vi "think_and_act.vi"(8 "error in (no error)":errorcluster, 9 "antState":T1, 10 "pieceOfWorld":T4[][](array[typedef]), 11 "Igor in":refnum<class "Igor.lvclass">) -> (0 "error out":errorcluster, 2 "action":T2, 3 "Igor out":refnum<class "Igor.lvclass">)   [LabVIEW 2015, in "Igor.lvclass"]
doc: "Ant thinks and chooses action\nCreated by Artem Shevelev\nshevelev.pro\nartem@shevelev.pro\nLabVIEW Portal: https://labviewportal.org/memberlist.php?mode=viewprofile&u=2340"
uses:
  Igor.lvclass
  actors/world/typedefs/worldCell_cluster.ctl
  actors/world/typedefs/markValue_cluster.ctl
  actors/world/typedefs/markValue.ctl
  actors/world/typedefs/markVolume.ctl
  actors/world/typedefs/amountOfFood.ctl
  actors/world/typedefs/anthillType_enum.ctl
  ant_base/action_cluster.ctl
  ant_base/actionType_enum.ctl
  ant_base/antState_cluster.ctl
  ant_base/ant_base.lvclass/ant_base.ctl
  ant_base/memory_limit_const.vi
  moving/move_forvard.vi
  moving/move_back.vi
  ant_base/ant_base.lvclass
  actors/world/world.lvlib
panel:
  out "Array":i32[][](array[numeric])
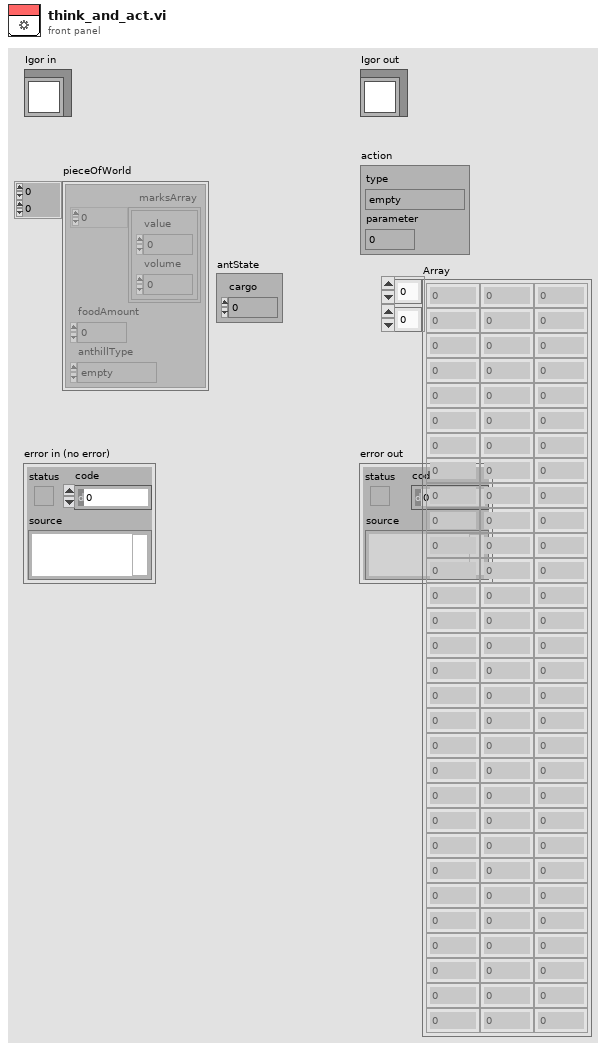
[diagram p1: front panel]
types:
  T1 = typedef "ant_base.lvclass/antState_cluster.ctl" = cluster{"cargo":u8}
  T2 = typedef "ant_base.lvclass/action_cluster.ctl" = cluster{"type":T3, "parameter":dbl}
  T3 = typedef "ant_base.lvclass/actionType_enum.ctl" = enum8{"empty", "move", "take", "put", "mark"}
  T4 = typedef "world.lvlib/worldCell_cluster.ctl" = cluster{"marksArray":T5[], "foodAmount":T8, "anthillType":T9}
  T5 = typedef "world.lvlib/markValue_cluster.ctl" = cluster{"value":T6, "volume":T7}
  T6 = typedef "world.lvlib/markValue.ctl" = u8
  T7 = typedef "world.lvlib/markVolume.ctl" = u16
  T8 = typedef "world.lvlib/amountOfFood.ctl" = i32
  T9 = typedef "world.lvlib/anthillType_enum.ctl" = enum16{"empty", "own", "rival"}
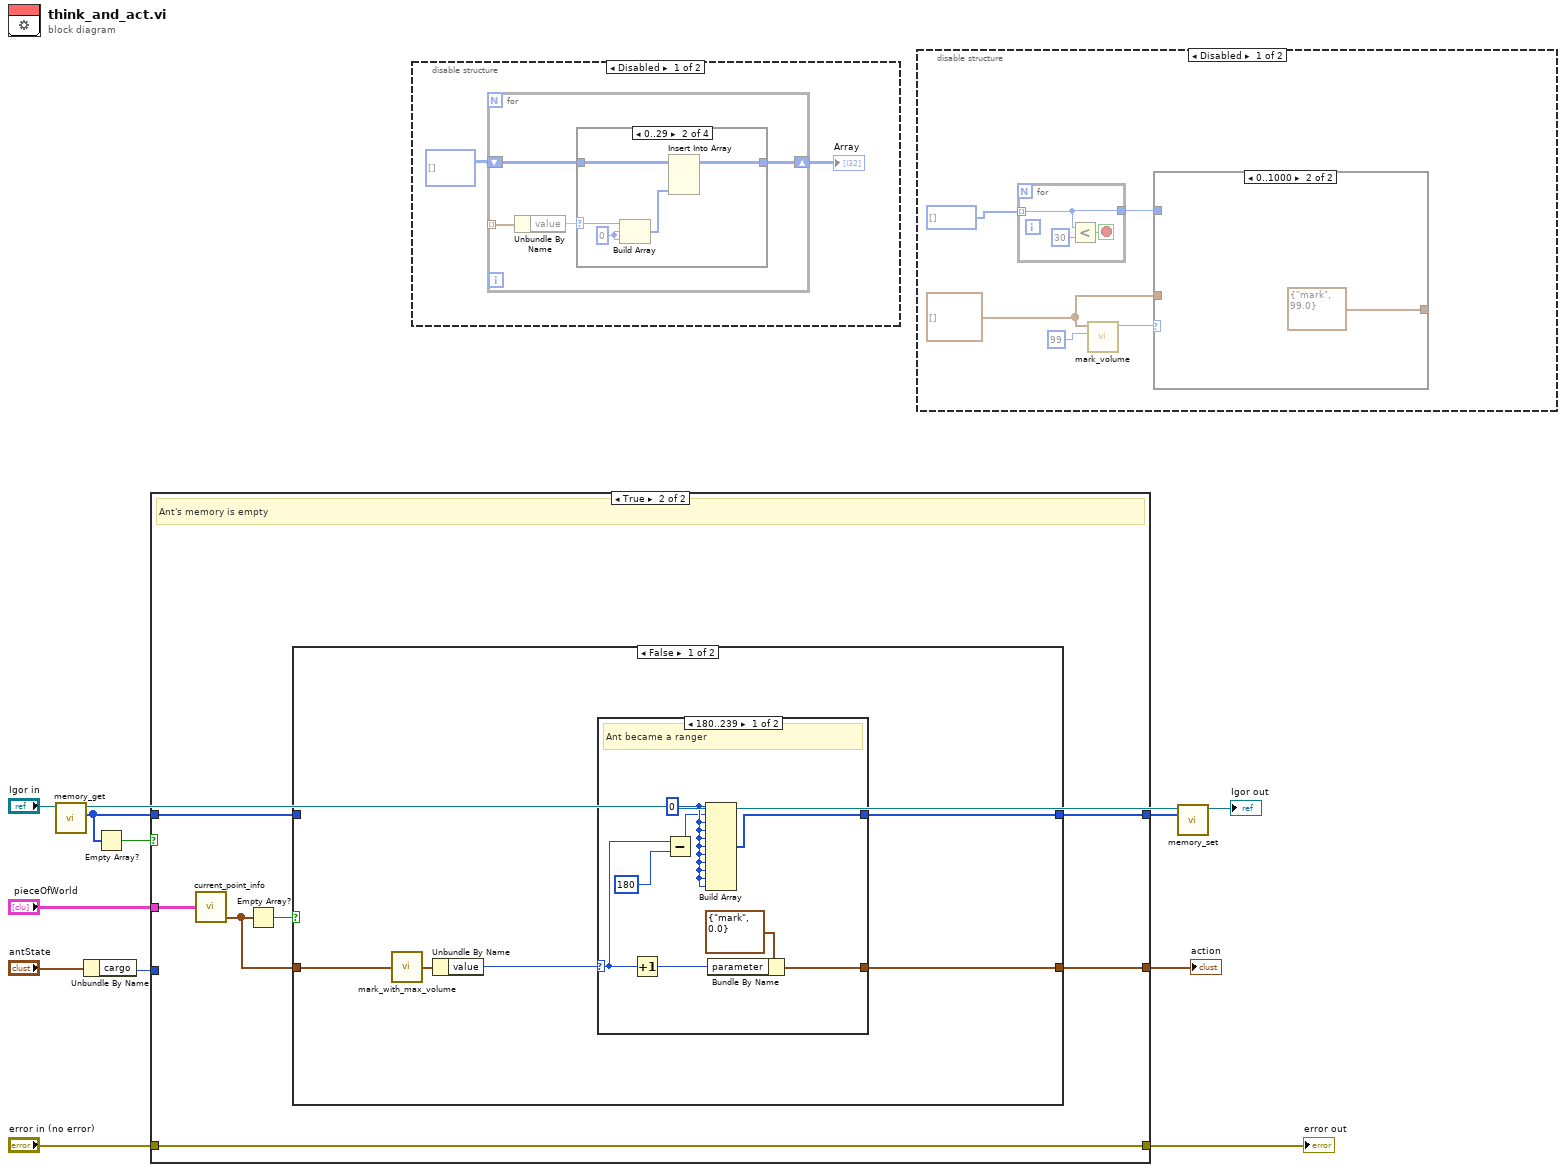
[diagram p0: block diagram]
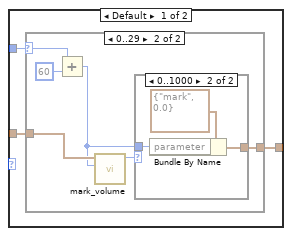
[diagram p2: hidden frame]
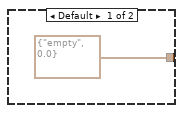
[diagram p3: hidden frame]
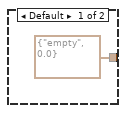
[diagram p4: hidden frame]
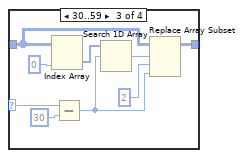
[diagram p7: hidden frame]
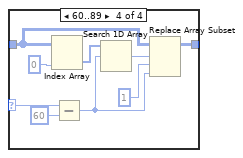
[diagram p8: hidden frame]
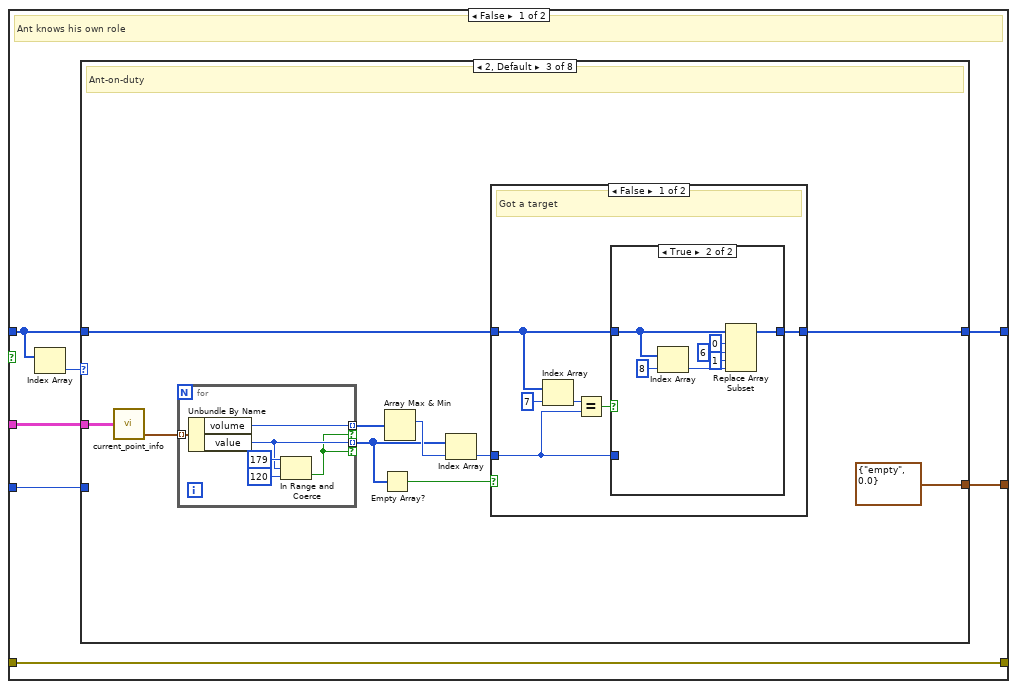
[diagram p10: hidden frame]
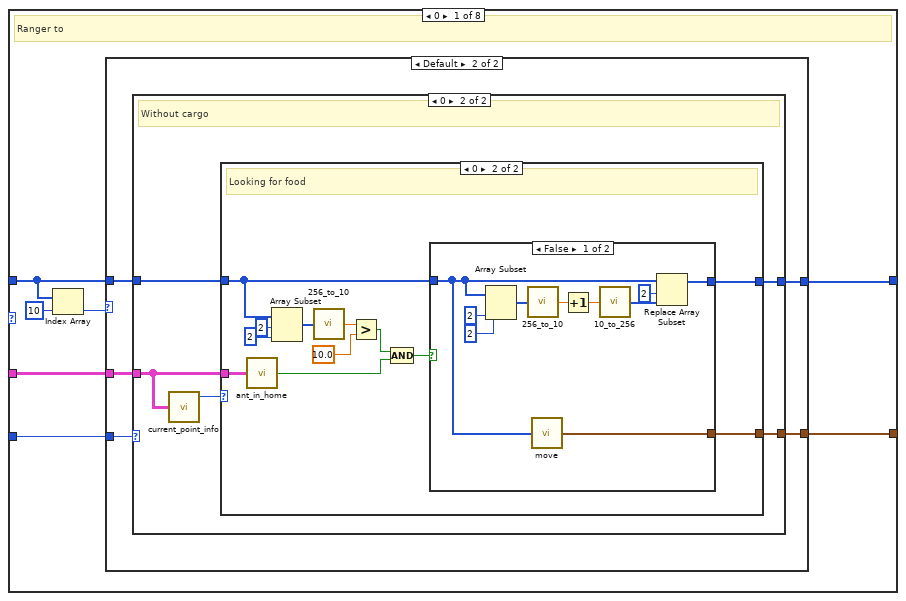
[diagram p11: hidden frame]
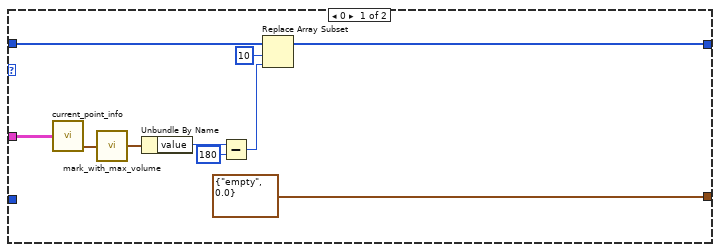
[diagram p12: hidden frame]
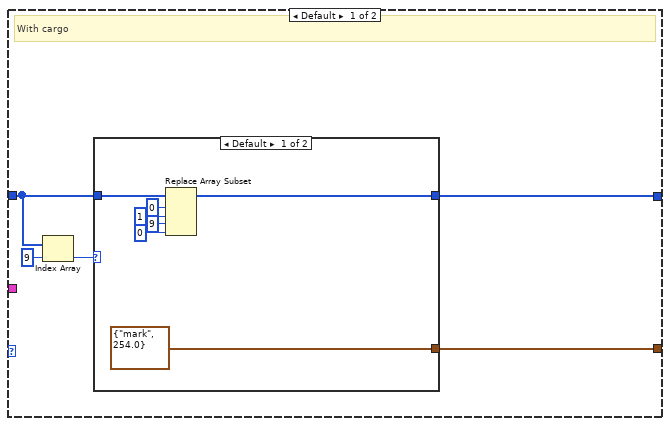
[diagram p13: hidden frame]
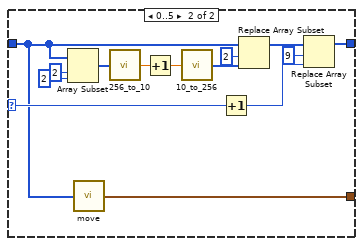
[diagram p14: hidden frame]
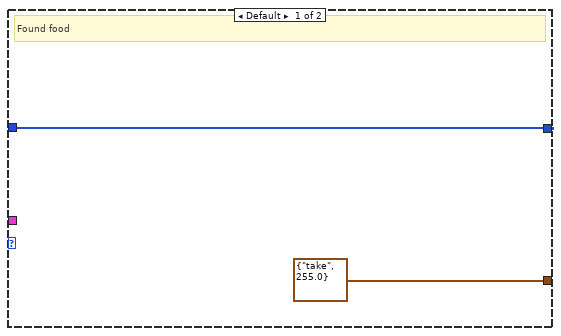
[diagram p15: hidden frame]
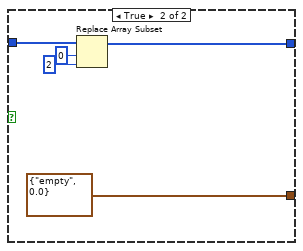
[diagram p16: hidden frame]
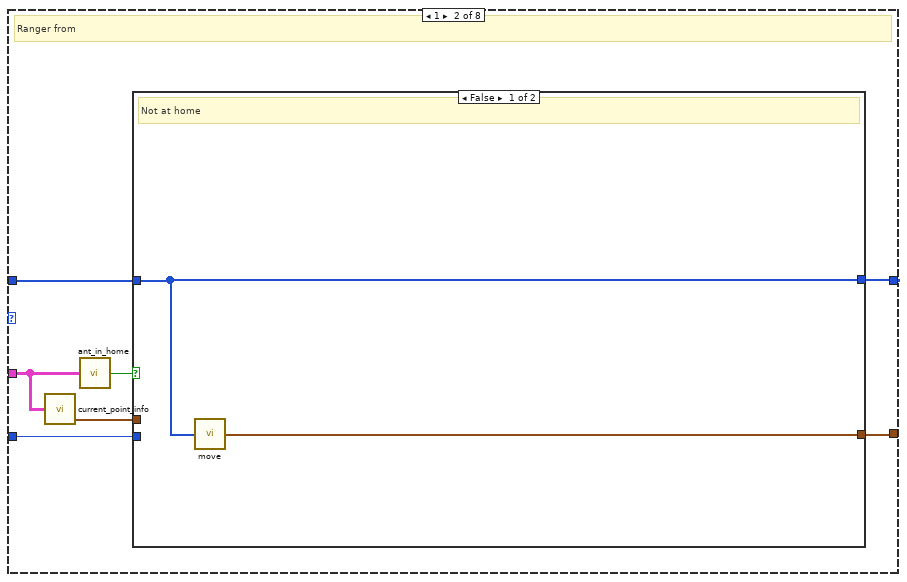
[diagram p17: hidden frame]
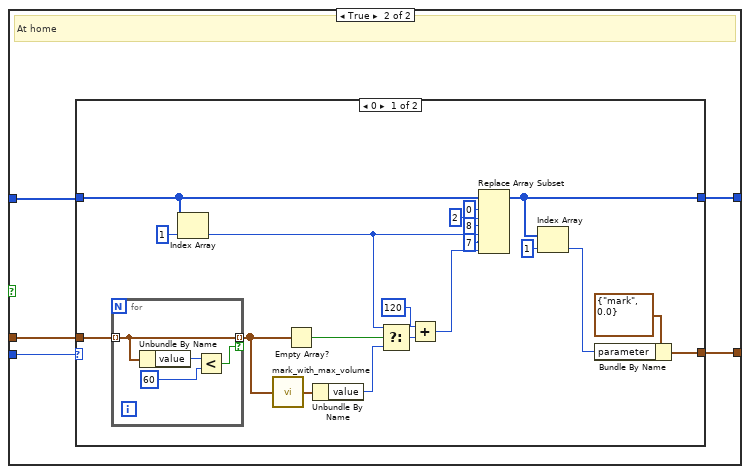
[diagram p18: hidden frame]
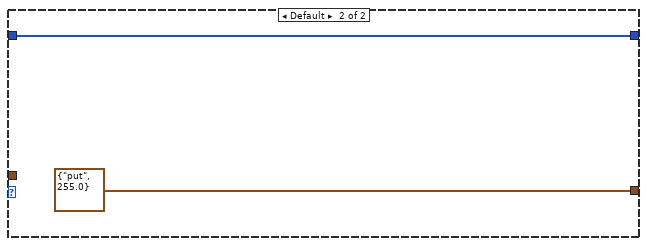
[diagram p19: hidden frame]
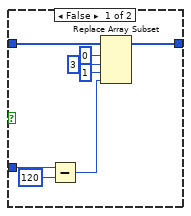
[diagram p20: hidden frame]
diagram:
  n1 = call "memory_get.vi"("ant_base in"="Igor in") -> ("memory"=w2:u8[], "ant_base out"=w7:refnum<class "Igor.lvclass">)  [unwired: 8 in, 1 out]
  n2 = Unbundle By Name("antState") -> ("cargo"=w3:u8)
  n3 = Empty Array?(array=w2) -> (empty?=w9:bool)
  n4 = case shown="True" w9 {
    tunnel: [w19 w390] -> w4
    tunnel: [w17 w389] -> w12
    tunnel: "error in (no error)" -> [w19 w390]
    tunnel: w2 -> [w16 w386]
    tunnel: "pieceOfWorld" -> [w15 w385]
    tunnel: [w14 w387] -> w6
    tunnel: w3 -> [w13 _]
    frame False {
      # "Ant knows his own role"
      n5 = Index Array(array=w16) -> (element=w18:u8)  [unwired: 1 in]
      n6 = case shown="2, Default" w18 {
        tunnel: [w26 w108 T2 {"type"=enum."empty", "parameter"=0.0} ("action") w190 w225 w243 w294 w329] -> w17
        tunnel: w16 -> [w22 w107 w144 w191 w224 w246 w295 w328]
        tunnel: w15 -> [w23 w103 w143 w181 w222 w242 w291 w326]
        tunnel: [w25 w106 w147 w188 w223 w244 w293 w327] -> w14
        tunnel: w13 -> [w24 w105 _ _ _ w247 _ _]
        frame 0 {
          # "Ranger to"
          n7 = Index Array(array=w22, index=10) -> (element=w20:u8)
          n8 = case shown="Default" w20 {
            tunnel: [T2 {"type"=enum."empty", "parameter"=0.0} ("action") w41] -> w26
            tunnel: w22 -> [w30 w40]
            tunnel: [w29 w39] -> w25
            tunnel: w24 -> [_ w38]
            tunnel: w23 -> [w35 w37]
            frame 0 {
              n9 = call "current_point_info.vi"("pieceOfWorld"=w35) -> ("marksArray"=w34:T5[])  [unwired: 2 out]
              n10 = call "mark_with_max_volume.vi"("marksArray"=w34) -> ("markValue"=w33:T5)
              n11 = Unbundle By Name(w33) -> ("value"=w32:T6)
              n12 = Subtract(x=w32, y=T6 180) -> (x-y=w28:T6)
              n13 = Replace Array Subset(array=w30, new element=w28, index=10) -> (w29:u8[])
            }
            frame Default {
              n14 = case shown="0" w38 {
                tunnel: [w45 w72] -> w41
                tunnel: w40 -> [w44 w71]
                tunnel: [w46 w70] -> w39
                tunnel: w37 -> [_ w69]
                frame Default {
                  # "With cargo"
                  n15 = Index Array(array=w44, index=9) -> (element=w42:u8)
                  n16 = case shown="Default" w42 {
                    selector: w42 -> [_ w65]
                    tunnel: [w50 w67] -> w46
                    tunnel: w44 -> [w51 w55]
                    tunnel: [T2 {"type"=enum."mark", "parameter"=254.0} ("action") w54] -> w45
                    frame Default {
                      n17 = Replace Array Subset(array=w51, new element #1=u8 1 ("new element/subarray"), index #1=0 ("index"), new element #2=u8 0 ("new element/subarray"), index #2=9 ("index")) -> (w50:u8[])
                    }
                    frame 0..5 {
                      n18 = Array Subset(array=w55, index=2, length=2) -> (w60:u8[])
                      n19 = call-poly "move.vi"("Ant's memory"=w55) -> ("action"=w54:T2)
                      n20 = call "256_to_10.vi"("Array"=w60) -> ("Numeric"=w59:dbl)
                      n21 = Increment(x=w59) -> (x+1=w58:dbl)
                      n22 = call "10_to_256.vi"("Decimal"=w58) -> ("256"=w57:u8[])
                      n23 = Increment(x=w65) -> (x+1=w64:u8)
                      n24 = Replace Array Subset(array=w55, new element=w57, index=2) -> (w56:u8[])
                      n25 = Replace Array Subset(array=w56, new element=w64, index=9) -> (w67:u8[])
                    }
                  }
                }
                frame 0 {
                  # "Without cargo"
                  n26 = call "current_point_info.vi"("pieceOfWorld"=w69) -> ("foodAmount"=w68:T8)  [unwired: 2 out]
                  n27 = case shown="0" w68 {
                    tunnel: [T2 {"type"=enum."take", "parameter"=255.0} ("action") w86] -> w72
                    tunnel: w71 -> [w73 w81]
                    tunnel: [w73 w85] -> w70
                    tunnel: w69 -> [_ w76]
                    frame Default {
                      # "Found food"
                    }
                    frame 0 {
                      # "Looking for food"
                      n28 = call "ant_in_home.vi"("pieceOfWorld"=w76) -> ("x .and. y?"=w75:bool)
                      n29 = Array Subset(array=w81, index=2, length=2) -> (w82:u8[])
                      n30 = call "256_to_10.vi"("Array"=w82) -> ("Numeric"=w80:dbl)
                      n31 = Greater?(x=w80, y=10.0) -> (0:w78:bool)
                      n32 = Compound Arithmetic op=AND(w78, w75) -> (w77:bool)
                      n33 = case shown="False" w77 {
                        tunnel: [w87 T2 {"type"=enum."empty", "parameter"=0.0} ("action")] -> w86
                        tunnel: [w89 w100] -> w85
                        tunnel: w81 -> [w88 w101]
                        frame False {
                          n34 = Array Subset(array=w88, index=2, length=2) -> (w93:u8[])
                          n35 = call "256_to_10.vi"("Array"=w93) -> ("Numeric"=w92:dbl)
                          n36 = call-poly "move.vi"("Ant's memory"=w88) -> ("action"=w87:T2)
                          n37 = Increment(x=w92) -> (x+1=w91:dbl)
                          n38 = call "10_to_256.vi"("Decimal"=w91) -> ("256"=w90:u8[])
                          n39 = Replace Array Subset(array=w88, new element=w90, index=2) -> (w89:u8[])
                        }
                        frame True {
                          n40 = Replace Array Subset(array=w101, new element=u8 2 ("new element/subarray"), index=0) -> (w100:u8[])
                        }
                      }
                    }
                  }
                }
              }
            }
          }
        }
        frame 1 {
          # "Ranger from"
          n41 = call "current_point_info.vi"("pieceOfWorld"=w103) -> ("marksArray"=w102:T5[])  [unwired: 2 out]
          n42 = call "ant_in_home.vi"("pieceOfWorld"=w103) -> ("x .and. y?"=w104:bool)
          n43 = case shown="False" w104 {
            tunnel: [w109 w115] -> w108
            tunnel: w102 -> [_ w111]
            tunnel: w107 -> [w110 w114]
            tunnel: [w110 w113] -> w106
            tunnel: w105 -> [_ w112]
            frame False {
              # "Not at home"
              n44 = call-poly "move.vi"("Ant's memory"=w110) -> ("action"=w109:T2)
            }
            frame True {
              # "At home"
              n45 = case shown="0" w112 {
                tunnel: [w135 T2 {"type"=enum."put", "parameter"=255.0} ("action")] -> w115
                tunnel: w114 -> [w132 w140]
                tunnel: [w119 w140] -> w113
                tunnel: w111 -> [w128 _]
                frame 0 {
                  n46 = for {
                    tunnel: w128 -> [w139] mode=indexing
                    tunnel: [w139] -> w127 mode=indexing if=w136
                    n47 = Unbundle By Name(w139) -> ("value"=w138:T6)
                    n48 = Less?(x=w138, y=T6 60) -> (x < y?=w136:bool)
                  }
                  n49 = Index Array(array=w132, index=1) -> (element=w116:u8)
                  n50 = call "mark_with_max_volume.vi"("marksArray"=w127) -> ("markValue"=w124:T5)
                  n51 = Empty Array?(array=w127) -> (empty?=w123:bool)
                  n52 = Unbundle By Name(w124) -> ("value"=w121:T6)
                  n53 = Select(t=w116, s=w123, f=w121) -> (s? t:f=w122:T6)
                  n54 = Add(x=T6 120 ("y"), y=w122) -> (x+y=w117:T6)
                  n55 = Replace Array Subset(array=w132, new element #1=u8 2 ("new element/subarray"), index #1=0 ("index"), new element #2=w116, index #2=8 ("index"), new element #3=w117, index #3=7 ("index")) -> (w119:u8[])
                  n56 = Index Array(array=w119, index=1) -> (element=w118:u8)
                  n57 = Bundle By Name(cluster=T2 {"type"=enum."mark", "parameter"=0.0} ("action"), "parameter"=w118) -> (w135:T2)
                }
                frame Default {
                }
              }
            }
          }
        }
        frame 2, Default {
          # "Ant-on-duty"
          n58 = call "current_point_info.vi"("pieceOfWorld"=w143) -> ("marksArray"=w142:T5[])  [unwired: 2 out]
          n59 = for {
            tunnel: w142 -> [w155] mode=indexing
            tunnel: [w153] -> w146 mode=indexing if=w152
            tunnel: [w154] -> w150 mode=indexing if=w152
            n60 = Unbundle By Name(w155) -> ("volume"=w154:T7, "value"=w153:T6)
            n61 = In Range and Coerce(upper limit=T6 179, x=w153, lower limit=T6 120) -> (In Range?=w152:bool)  [unwired: 1 out]
          }
          n62 = Empty Array?(array=w146) -> (empty?=w145:bool)
          n63 = Array Max & Min(array=w150) -> (max index (indices)=w148:i32)  [unwired: 3 out]
          n64 = Index Array(array=w146, index=w148) -> (element=w149:T6)
          n65 = case shown="False" w145 {
            tunnel: w149 -> [w159 _]
            tunnel: w144 -> [w162 w179]
            tunnel: [w163 w179] -> w147
            frame False {
              # "Got a target"
              n66 = Index Array(array=w162, index=7) -> (element=w160:u8)
              n67 = Equal?(x=w160, y=w159) -> (x = y?=w158:bool)
              n68 = case shown="True" w158 {
                tunnel: w159 -> [w171 _]
                tunnel: w162 -> [w169 w173]
                tunnel: [w164 w175] -> w163
                frame False {
                  n69 = Subtract(x=w171, y=T6 120) -> (x-y=w165:T6)
                  n70 = Replace Array Subset(array=w169, new element #1=u8 3 ("new element/subarray"), index #1=0 ("index"), new element #2=w165, index #2=1 ("index")) -> (w164:u8[])
                }
                frame True {
                  n71 = Index Array(array=w173, index=8) -> (element=w172:u8)
                  n72 = Replace Array Subset(array=w173, new element #1=u8 6 ("new element/subarray"), index #1=0 ("index"), new element #2=w172, index #2=1 ("index")) -> (w175:u8[])
                }
              }
            }
            frame True {
              # "Expecting a target"
            }
          }
        }
        frame 3 {
          # "Worker without cargo"
          n73 = call "current_point_info.vi"("pieceOfWorld"=w181) -> ("foodAmount"=w180:T8)  [unwired: 2 out]
          n74 = Reshape Array(w181, 9 ("dimension size")) -> (w186:T4[])
          n75 = for {
            tunnel: w186 -> [w194] mode=indexing
            tunnel: [w193] -> w183 mode=concatenating
            tunnel: [w192] -> w185 mode=indexing
            n76 = Unbundle By Name(w194) -> ("foodAmount"=w192:T8, "marksArray"=w193:T5[])
          }
          n77 = Add Array Elements(numeric array=w185) -> (sum=w184:T8)
          n78 = call "mark_volume.vi"("element"=T6 254, "marksArray"=w183) -> ("volume"=w182:T7)  [unwired: 9 in]
          n79 = case shown="Default" w180 {
            tunnel: [T2 {"type"=enum."take", "parameter"=255.0} ("action") w204] -> w190
            tunnel: w191 -> [w198 w202]
            tunnel: w182 -> [_ w203]
            tunnel: [w195 w201] -> w188
            tunnel: w184 -> [_ w200]
            frame Default {
              # "Found a lot of food"
              n80 = Replace Array Subset(array=w198, new element=4 ("index"), index=0) -> (w195:u8[])
            }
            frame 0 {
              # "Looking for food"
              n81 = case shown="0" w203 {
                tunnel: [w205 T2 {"type"=enum."empty", "parameter"=0.0} ("action")] -> w204
                tunnel: w202 -> [w206 w213]
                tunnel: [w206 w212] -> w201
                tunnel: w200 -> [_ w211]
                frame 0 {
                  n82 = call-poly "move.vi"("Ant's memory"=w206) -> ("action"=w205:T2)
                }
                frame Default {
                  n83 = Equal To 0?(x=w211) -> (x = 0?=w210:bool)
                  n84 = Index Array(array=w213, index=1) -> (element=w215:u8)
                  n85 = Add(x=w215, y=u8 60) -> (x+y=w209:u8)
                  n86 = Select(t=w209, s=w210, f=u8 0) -> (s? t:f=w207:u8)
                  n87 = Replace Array Subset(array=w213, new element #1=u8 4 ("new element/subarray"), index #1=0 ("index"), new element #2=w207, index #2=6 ("index")) -> (w212:u8[])
                }
              }
            }
          }
        }
        frame 4 {
          # "Worker with cargo"
          n88 = call "ant_in_home.vi"("pieceOfWorld"=w222) -> ("x .and. y?"=w221:bool)
          n89 = case shown="True" w221 {
            tunnel: [w226 w235] -> w225
            tunnel: w224 -> [w227 w234]
            tunnel: [w227 w229] -> w223
            frame False {
              # "Not at home"
              n90 = call-poly "move.vi"("Ant's memory"=w227) -> ("action"=w226:T2)
            }
            frame True {
              # "At home"
              n91 = Index Array(array=w234, index=6) -> (element=w228:u8)
              n92 = case shown="60..119" w228 {
                selector: w228 -> [w237 _]
                tunnel: [w238 T2 {"type"=enum."put", "parameter"=255.0} ("action")] -> w235
                frame 60..119 {
                  n93 = Bundle By Name(cluster=T2 {"type"=enum."mark", "parameter"=0.0} ("action"), "parameter"=w237) -> (w238:T2)
                }
                frame Default {
                }
              }
              n94 = Replace Array Subset(array=w234, new element #1=u8 2 ("y"), index #1=0 ("index"), new element #2=u8 0 ("new element/subarray"), index #2=6 ("index")) -> (w229:u8[])
            }
          }
        }
        frame 6 {
          # "Expirienced ranger to foodHeap"
          n95 = call "current_point_info.vi"("pieceOfWorld"=w242) -> ("foodAmount"=w241:T8)  [unwired: 2 out]
          n96 = Array Subset(array=w246, index=2, length=2 ("index")) -> (w251:u8[])
          n97 = Array Subset(array=w246, index=4, length=2) -> (w253:u8[])
          n98 = call "256_to_10.vi"("Array"=w253) -> ("Numeric"=w250:dbl)
          n99 = call "256_to_10.vi"("Array"=w251) -> ("Numeric"=w248:dbl)
          n100 = Greater Or Equal?(x=w250, y=w248) -> (x >= y?=w245:bool)
          n101 = case shown="False" w245 {
            tunnel: w247 -> [w260 w278]
            tunnel: w241 -> [w261 _]
            tunnel: w246 -> [w263 w284]
            tunnel: [w256 T2 {"type"=enum."mark", "parameter"=254.0} ("action")] -> w243
            tunnel: [w262 w285] -> w244
            frame False {
              n102 = Greater Than 0?(x=w260) -> (x > 0?=w258:bool)
              n103 = Greater Than 0?(x=w261) -> (x > 0?=w259:bool)
              n104 = Implies(1:w258, 2:w259) -> (0:w257:bool)
              n105 = case shown="True" w257 {
                tunnel: [w264 w275] -> w262
                tunnel: w263 -> [w264 w267]
                tunnel: [T2 {"type"=enum."take", "parameter"=255.0} ("action") w266] -> w256
                frame False {
                  # "Found food"
                }
                frame True {
                  # "No food in cell"
                  n106 = Array Subset(array=w267, index=4, length=2) -> (w271:u8[])
                  n107 = call-poly "move.vi"("Ant's memory"=w267) -> ("action"=w266:T2)
                  n108 = call "256_to_10.vi"("Array"=w271) -> ("Numeric"=w270:dbl)
                  n109 = Increment(x=w270) -> (x+1=w269:dbl)
                  n110 = call "10_to_256.vi"("Decimal"=w269) -> ("256"=w268:u8[])
                  n111 = Replace Array Subset(array=w267, new element=w268, index=4) -> (w275:u8[])
                }
              }
            }
            frame True {
              n112 = Less?(x=w278, y=u8 255) -> (x < y?=w276:bool)
              n113 = Index Array(array=w284) -> (element=w283:u8)  [unwired: 1 in]
              n114 = Add(x=w283, y=u8 60) -> (x+y=w281:u8)
              n115 = Select(t=w281, s=w276, f=u8 0) -> (s? t:f=w279:u8)
              n116 = Replace Array Subset(array=w284, new element #1=u8 7 ("new element/subarray"), index #1=0 ("index"), new element #2=w279, index #2=6 ("index")) -> (w285:u8[])
            }
          }
        }
        frame 7 {
          # "Expirienced ranger from foodHeap"
          n117 = call "current_point_info.vi"("pieceOfWorld"=w291) -> ("marksArray"=w290:T5[])  [unwired: 2 out]
          n118 = call "ant_in_home.vi"("pieceOfWorld"=w291) -> ("x .and. y?"=w292:bool)
          n119 = case shown="True" w292 {
            tunnel: [w296 w306] -> w294
            tunnel: w295 -> [w297 w303]
            tunnel: [w297 w305] -> w293
            tunnel: w290 -> [_ w304]
            frame False {
              # "Not at home"
              n120 = call-poly "move.vi"("Ant's memory"=w297) -> ("action"=w296:T2)
            }
            frame True {
              # "At home"
              n121 = Index Array(array=w303, index=1) -> (element=w298:u8)
              n122 = Add(x=w298, y=u8 60) -> (x+y=w300:u8)
              n123 = call "mark_volume.vi"("element"=w300, "marksArray"=w304) -> ("volume"=w299:T7)  [unwired: 9 in]
              n124 = case shown="Default" w299 {
                tunnel: [T2 {"type"=enum."put", "parameter"=255.0} ("action") T2 {"type"=enum."put", "parameter"=255.0} ("action")] -> w306
                tunnel: w303 -> [w309 w320]
                tunnel: [w313 w318] -> w305
                tunnel: w298 -> [w312 _]
                frame Default {
                  w310 = u8 0 ("y")
                  n125 = Index Array(array=w309, index=10) -> (element=w307:u8)
                  n126 = Build Array(w310, w312, w310, w310, w310, w310, w310, w310, w310, w310, w307) -> (w313:u8[])
                }
                frame 0 {
                  n127 = Replace Array Subset(array=w320, new element #1=u8 6 ("new element/subarray"), index #1=0 ("index"), new element #2=u8 0 ("new element/subarray"), index #2=4 ("index"), new element #3=u8 0 ("new element/subarray"), index #3=5 ("index")) -> (w318:u8[])
                }
              }
            }
          }
        }
        frame 180 {
          # "Administrator"
          n128 = call "current_point_info.vi"("pieceOfWorld"=w326) -> ("marksArray"=w325:T5[])  [unwired: 2 out]
          n129 = for {
            tunnel: w325 -> [w354] mode=indexing
            shift-right: [w352] -> w327
            shift-left: w328 -> [w353]
            n130 = Unbundle By Name(w354) -> ("value"=w351:T6)
            n131 = case shown="0..59" w351 {
              selector: w351 -> [_ w360 w373]
              tunnel: w353 -> [w355 w361 w375]
              tunnel: [w355 w358 w374] -> w352
              frame Default {
              }
              frame 0..59 {
                n132 = Add(x=w360, y=T6 60) -> (x+y=w363:T6)
                n133 = Search 1D Array(1D array=w361, element=w360) -> (index of element=w356:i32)  [unwired: 1 in]
                n134 = Search 1D Array(1D array=w361, element=w363) -> (index of element=w357:i32)  [unwired: 1 in]
                n135 = case shown="-1" w356 {
                  tunnel: w361 -> [w368 w371]
                  tunnel: [w368 w370] -> w359
                  tunnel: w360 -> [_ w369]
                  frame Default {
                  }
                  frame -1 {
                    n136 = Insert Into Array(array=w371, new element=w369) -> (w370:u8[])  [unwired: 1 in]
                  }
                }
                n137 = case shown="Default" w357 {
                  selector: w357 -> [_ w365]
                  tunnel: w359 -> [w364 w367]
                  tunnel: [w364 w366] -> w358
                  frame -1 {
                  }
                  frame Default {
                    n138 = Delete From Array(array=w367, index=w365) -> (array with subset deleted=w366:u8[])  [unwired: 1 in, 1 out]
                  }
                }
              }
              frame 60..119 {
                n139 = Search 1D Array(1D array=w375, element=w373) -> (index of element=w372:i32)  [unwired: 1 in]
                n140 = case shown="-1" w372 {
                  tunnel: w375 -> [w376 w381]
                  tunnel: [w376 w379] -> w374
                  tunnel: w373 -> [_ w378]
                  frame 0, Default {
                  }
                  frame -1 {
                    n141 = Subtract(x=w378, y=T6 60) -> (x-y=w383:T6)
                    n142 = Insert Into Array(array=w381, new element=w378) -> (w380:u8[])  [unwired: 1 in]
                    n143 = Search 1D Array(1D array=w381, element=w383) -> (index of element=w377:i32)  [unwired: 1 in]
                    n144 = Delete From Array(array=w380, index=w377) -> (array with subset deleted=w379:u8[])  [unwired: 1 in, 1 out]
                  }
                }
              }
            }
          }
          n145 = call "mark_volume.vi"("element"=T6 180, "marksArray"=w325) -> ("volume"=w323:T7)  [unwired: 9 in]
          n146 = case shown="Default" w323 {
            tunnel: [w332 T2 {"type"=enum."mark", "parameter"=180.0} ("action")] -> w329
            tunnel: w327 -> [w330 _]
            tunnel: w325 -> [w331 _]
            frame Default {
              n147 = for {
                tunnel: [w336] -> w332
                tunnel: w331 -> [w335]
                tunnel: w330 -> [w333] mode=indexing
                stop <- w334 stop-if-true
                n148 = case shown="0..59" w333 {
                  selector: w333 -> [_ w339]
                  tunnel: [T2 {"type"=enum."empty", "parameter"=0.0} ("action") w345] -> w336
                  tunnel: w335 -> [_ w344]
                  tunnel: [FALSE TRUE] -> w334
                  frame Default {
                  }
                  frame 0..59 {
                    n149 = Add(x=w339, y=u8 120) -> (x+y=w342:u8)
                    n150 = call "mark_volume.vi"("element"=w342, "marksArray"=w344) -> ("volume"=w341:T7)  [unwired: 9 in]
                    n151 = case shown="0..1000" w341 {
                      tunnel: [T2 {"type"=enum."empty", "parameter"=0.0} ("action") w349] -> w345
                      tunnel: w342 -> [_ w348]
                      frame Default {
                      }
                      frame 0..1000 {
                        n152 = Bundle By Name(cluster=T2 {"type"=enum."mark", "parameter"=0.0} ("action"), "parameter"=w348) -> (w349:T2)
                      }
                    }
                  }
                }
              }
            }
            frame 0..1000 {
            }
          }
        }
      }
    }
    frame True {
      # "Ant's memory is empty"
      n153 = call "current_point_info.vi"("pieceOfWorld"=w385) -> ("marksArray"=w384:T5[])  [unwired: 2 out]
      n154 = Empty Array?(array=w384) -> (empty?=w388:bool)
      n155 = case shown="False" w388 {
        tunnel: [w395 w416] -> w389
        tunnel: [w394 w414] -> w387
        tunnel: w386 -> [_ _]
        tunnel: w384 -> [w393 _]
        frame False {
          n156 = call "mark_with_max_volume.vi"("marksArray"=w393) -> ("markValue"=w392:T5)
          n157 = Unbundle By Name(w392) -> ("value"=w391:T6)
          n158 = case shown="180..239" w391 {
            selector: w391 -> [w397 w406]
            tunnel: [w402 w410] -> w395
            tunnel: [w401 w408] -> w394
            frame 180..239 {
              w400 = T6 0 ("element")
              # "Ant became a ranger"
              n159 = Increment(x=w397) -> (x+1=w399:T6)
              n160 = Subtract(x=w397, y=T6 180) -> (x-y=w396:T6)
              n161 = Build Array(w400, w396, w400, w400, w400, w400, w400, w400, w400, w400, w400) -> (w401:T6[])
              n162 = Bundle By Name(cluster=T2 {"type"=enum."mark", "parameter"=0.0} ("action"), "parameter"=w399) -> (w402:T2)
            }
            frame Default {
              w407 = T6 0 ("element")
              # "Ant became an ant-on-duty"
              n163 = Subtract(x=w406, y=T6 180) -> (x-y=w404:T6)
              n164 = Build Array(T6 2 ("element"), w407, w407, w407, w407, w407, w407, w407, w407, w407, w404) -> (w408:T6[])
              n165 = Bundle By Name(cluster=T2 {"type"=enum."mark", "parameter"=0.0} ("action"), "parameter"=w406) -> (w410:T2)
            }
          }
        }
        frame True {
          # "The very first ant"
          n166 = Build Array(T6 180 ("element")) -> (w414:T6[])
          n167 = Bundle By Name(cluster=T2 {"type"=enum."mark", "parameter"=0.0} ("action"), "parameter"=T6 180 ("element")) -> (w416:T2)
        }
      }
    }
  }
  "error out" <- w4
  "action" <- w12
  n168 = disable-structure shown="Disabled" {
    frame Disabled {
      n169 = for {
        tunnel: _ -> [w422] mode=indexing
        shift-right: [w419] -> w418
        shift-left: i32[][] [] -> [w420]
        n170 = Unbundle By Name(w422) -> ("value"=w421)
        n171 = case shown="0..29" w421 {
          selector: w421 -> [_ w426 w431 w440]
          tunnel: w420 -> [w423 w428 w435 w444]
          tunnel: [w423 w427 w432 w441] -> w419
          frame Default {
          }
          frame 0..29 {
            w425 = T6 0 ("element")
            n172 = Build Array(w426, w425, w425) -> (w424:T6[])
            n173 = Insert Into Array(array=w428, new element=w424) -> (w427:i32[][])  [unwired: 2 in]
          }
          frame 30..59 {
            n174 = Index Array(array=w435, index (col)=0 ("disabled index (col)")) -> (element=w436:i32[])  [unwired: 1 in]
            n175 = Subtract(x=w431, y=T6 30) -> (x-y=w429:T6)
            n176 = Search 1D Array(1D array=w436, element=w429) -> (index of element=w434:i32)  [unwired: 1 in]
            n177 = Replace Array Subset(array=w435, new element=w429, index (row)=w434, index (col)=2 ("disabled index (col)")) -> (w432:i32[][])
          }
          frame 60..89 {
            n178 = Index Array(array=w444, index (col)=0 ("disabled index (col)")) -> (element=w445:i32[])  [unwired: 1 in]
            n179 = Subtract(x=w440, y=T6 60) -> (x-y=w438:T6)
            n180 = Search 1D Array(1D array=w445, element=w438) -> (index of element=w443:i32)  [unwired: 1 in]
            n181 = Replace Array Subset(array=w444, new element=w438, index (row)=w443, index (col)=1 ("disabled index (col)")) -> (w441:i32[][])
          }
        }
      }
      "Array" <- w418
    }
    frame Enabled {
    }
  }
  n182 = disable-structure shown="Disabled" {
    frame Disabled {
      w448 = T5[] [] ("marksArray")
      n183 = for {
        tunnel: u8[] [] ("memory") -> [w469] mode=indexing
        tunnel: [w469] -> w451
        stop <- w467 stop-if-true
        n184 = Less?(x=w469, y=u8 30) -> (x < y?=w467:bool)
      }
      n185 = call "mark_volume.vi"("element"=T6 99, "marksArray"=w448) -> ("volume"=w449:T7)  [unwired: 9 in]
      n186 = case shown="0..1000" w449 {
        tunnel: [w454 T2 {"type"=enum."mark", "parameter"=99.0} ("action")] -> _
        tunnel: w451 -> [w452 _]
        tunnel: w448 -> [w453 _]
        frame Default {
          n187 = case shown="0..29" w452 {
            selector: w452 -> [_ w457]
            tunnel: [T2 {"type"=enum."empty", "parameter"=0.0} ("action") w461] -> w454
            tunnel: w453 -> [_ w460]
            frame Default {
            }
            frame 0..29 {
              n188 = Add(x=w457, y=u8 60) -> (x+y=w458:u8)
              n189 = call "mark_volume.vi"("element"=w458, "marksArray"=w460) -> ("volume"=w456:T7)  [unwired: 9 in]
              n190 = case shown="0..1000" w456 {
                tunnel: [T2 {"type"=enum."empty", "parameter"=0.0} ("action") w465] -> w461
                tunnel: w458 -> [_ w464]
                frame Default {
                }
                frame 0..1000 {
                  n191 = Bundle By Name(cluster=T2 {"type"=enum."mark", "parameter"=0.0} ("action"), "parameter"=w464) -> (w465:T2)
                }
              }
            }
          }
        }
        frame 0..1000 {
        }
      }
    }
    frame Enabled {
    }
  }
  n192 = call "memory_set.vi"("memory"=w6, "ant_base in"=w7) -> ("ant_base out"=→"Igor out":refnum<class "Igor.lvclass">)  [unwired: 8 in, 1 out]
